vi "Live Image Test_cpattern match.vi"() -> ()   [LabVIEW 2017]
uses:
  <vilib>/vision/NI_Vision_Development_Module.lvlib
panel:
  in  "Minimum Score":sgl=700.0
  in  "Learn":bool
  in  "Test":enum16{"Color Pattern", "no test"}(ring)
  in  "Enum":T1(ring)
  in  "Acquire Params":T2={"fps"=10, "Compression"=30, "X"=320, "Y"=240, "Enable Color?"=TRUE, "Rotation"=enum."0"}
  out "Waveform Chart":u32(graph)
  out "dT":u32
  in  "stop":bool
  out "Image":T3(plugin-control)
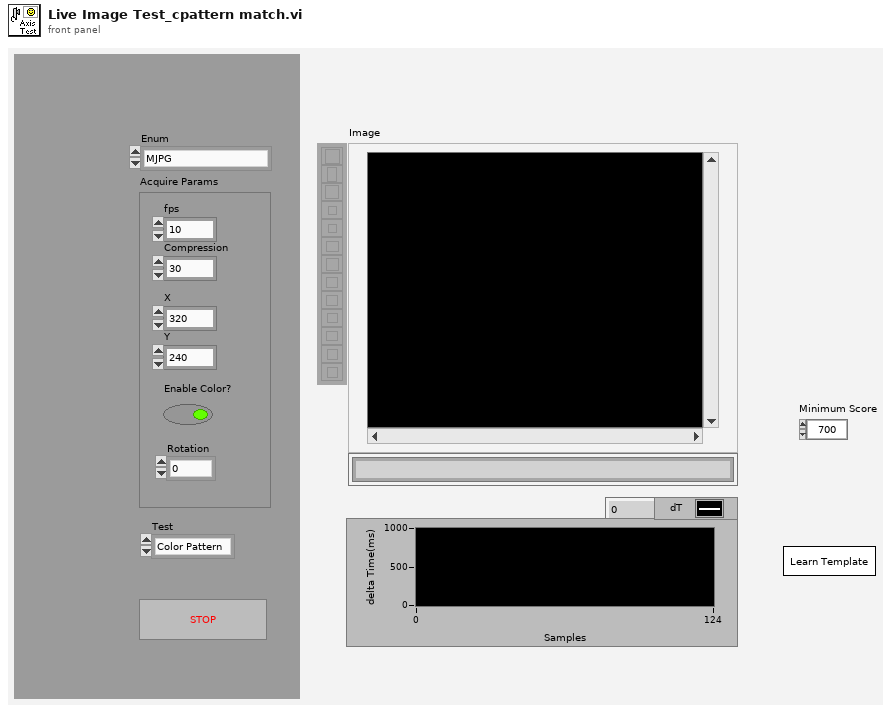
[diagram p1: front panel]
types:
  T1 = enum16{"MJPG", "JPG", "JPG-CGI", "BMP", "BMP-CGI"}
  T2 = cluster{"fps":i32, "Compression":i32, "X":i32, "Y":i32, "Enable Color?":bool, "Rotation":enum16{"0", "90", "180", "270"}}
  T3 = typedef "IMAQ Image.ctl" = refnum<image>
  T4 = typedef "Image Type" = u32
  T5 = cluster{"Global Rectangle":i32[], "Contours":cluster{"Contour Type":u32, "ROI Type":u32, "Points":i32[]}[]}
  T6 = cluster{i32[], cluster{"Contour Type":u32, "ROI Type":u32, i32[]}[]}
  T7 = cluster{"Position":cluster{"x":sgl, "y":sgl}, "Angle":sgl, "Scale":sgl, "Score":sgl, "Bounding Box":cluster{"x":sgl, "y":sgl}[]}[]
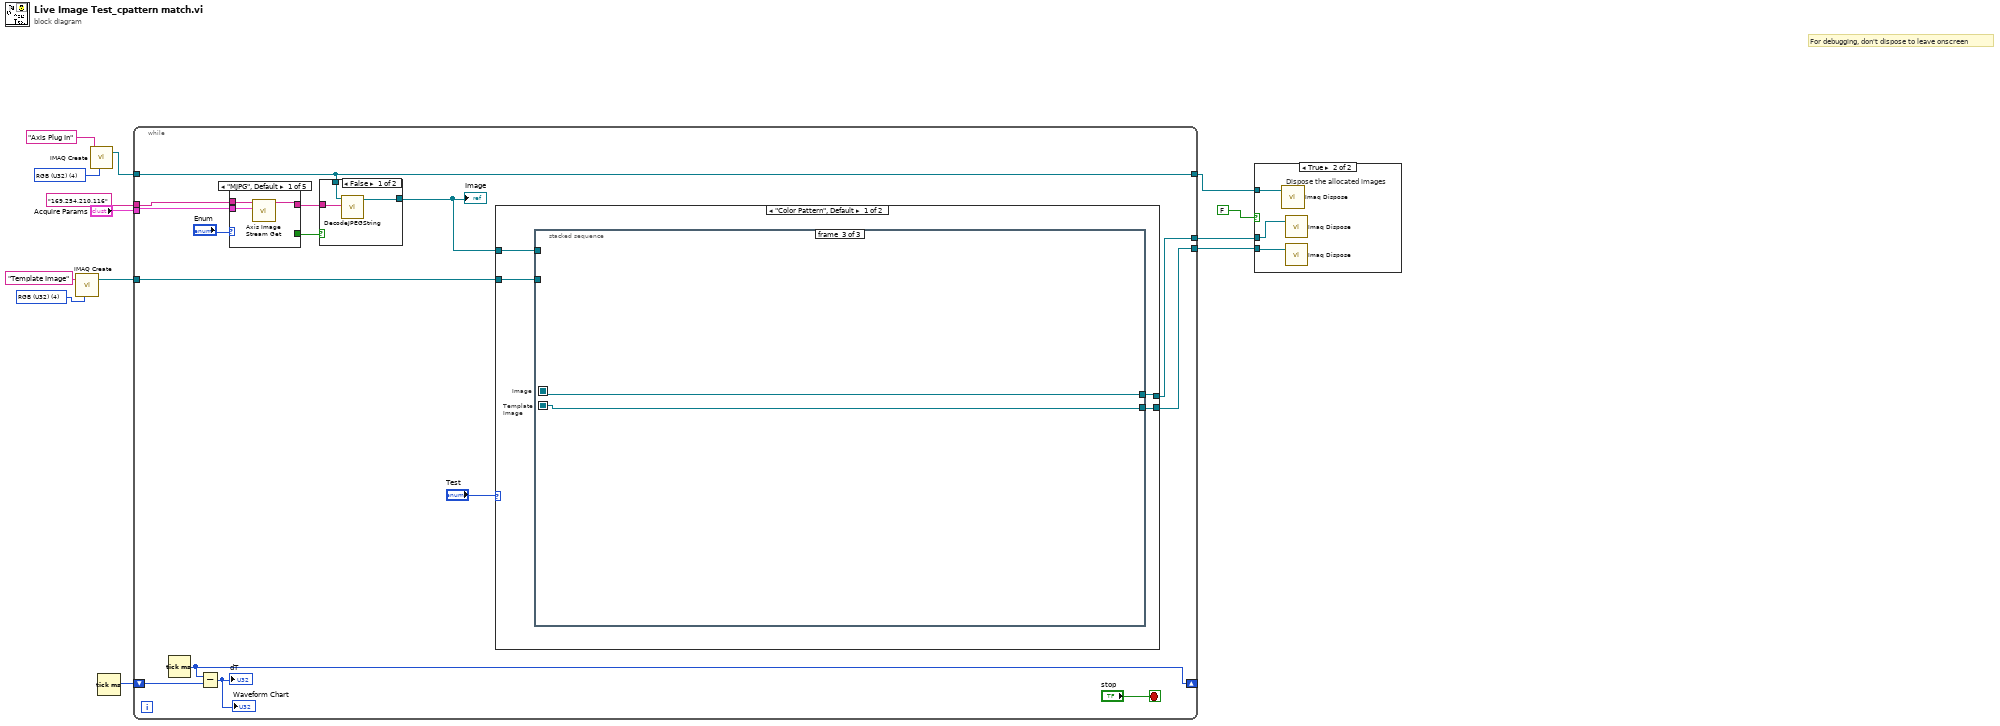
[diagram p0: block diagram]
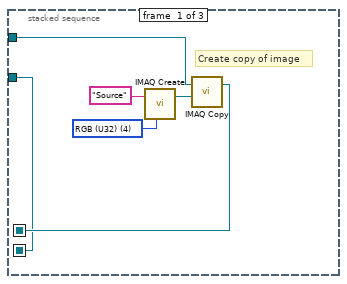
[diagram p3: hidden frame]
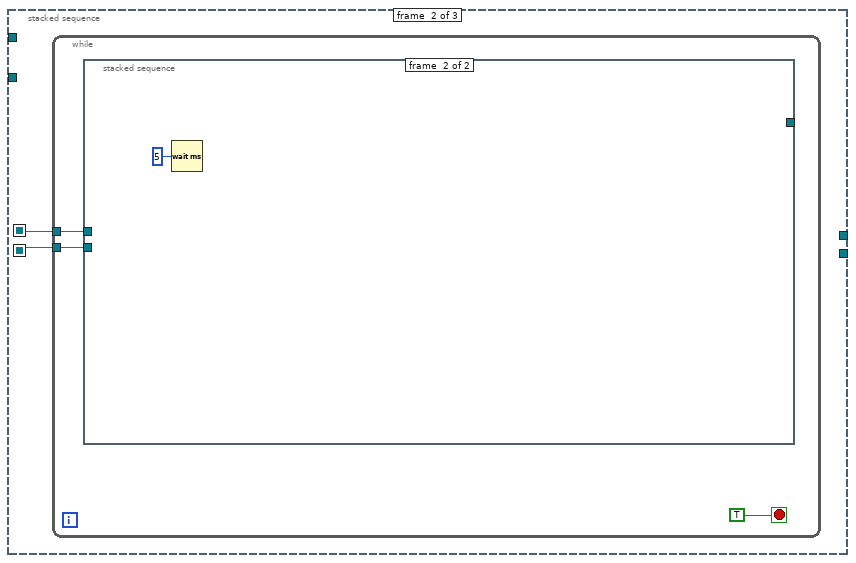
[diagram p4: hidden frame]
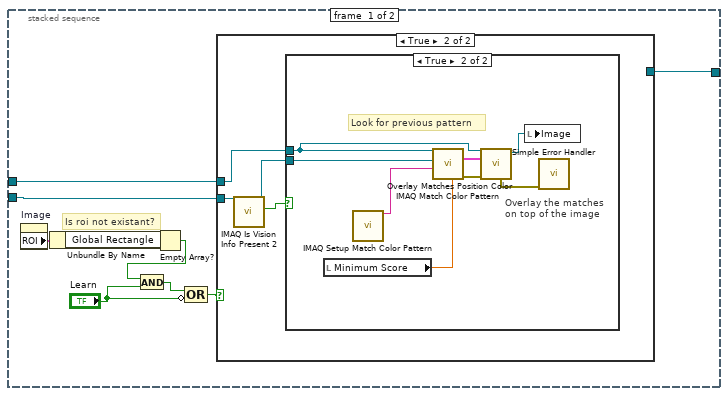
[diagram p5: hidden frame]
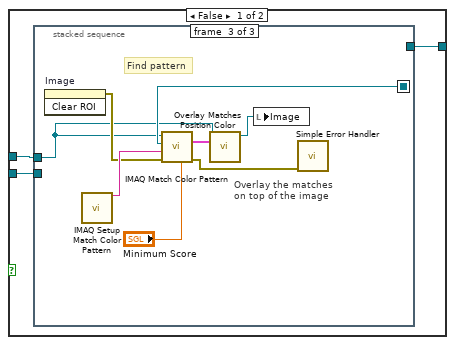
[diagram p6: hidden frame]
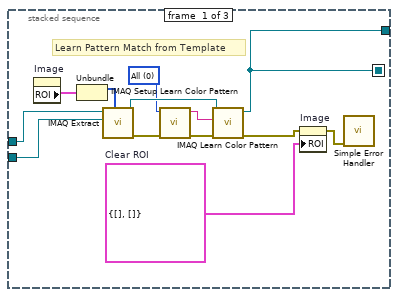
[diagram p7: hidden frame]
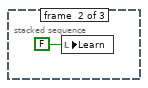
[diagram p8: hidden frame]
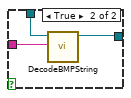
[diagram p11: hidden frame]
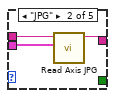
[diagram p12: hidden frame]
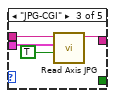
[diagram p13: hidden frame]
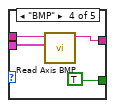
[diagram p14: hidden frame]
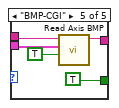
[diagram p15: hidden frame]
diagram:
  w5 = T4 4 items=["Grayscale (U8)", "Grayscale (I16)", "Grayscale (SGL)", "Complex (CSG)", "RGB (U32)", "HSL (U32)", "RGB (U64)", "Grayscale (U16)"] ("Image Type")
  w6 = T4 4 items=["Grayscale (U8)", "Grayscale (I16)", "Grayscale (SGL)", "Complex (CSG)", "RGB (U32)", "HSL (U32)", "RGB (U64)"] ("Image Type")
  # "For debugging, don't dispose to leave onscreen"
  n1 = call "IMAQ Create"("Image Name"="Template Image", "Image Type"=w5) -> ("New Image"=w3:T3)  [unwired: 3 in, 1 out]
  n2 = call "IMAQ Create"("Image Name"="Axis Plug In", "Image Type"=w6) -> ("New Image"=w12:T3)  [unwired: 3 in, 1 out]
  n3 = Tick Count (ms)() -> (millisecond timer value=w11:u32)
  n4 = while {
    tunnel: w12 -> [w24]
    shift-right: [w26] -> _
    shift-left: w11 -> [w27]
    tunnel: [w24] -> w10
    tunnel: "169.254.210.116" ("address") -> [w23]
    tunnel: "Acquire Params" -> [w20]
    tunnel: w3 -> [w17]
    tunnel: [w16] -> w2
    tunnel: [w15] -> w1
    stop <- "stop" stop-if-true
    n5 = Tick Count (ms)() -> (millisecond timer value=w26:u32)
    n6 = Subtract(x=w26, y=w27) -> (x-y=→"dT" →"Waveform Chart":u32)
    n7 = case shown="\"MJPG\", Default" "Enum" {
      tunnel: w23 -> [w100 w103 w107 w111 w115]
      tunnel: [w99 w102 w106 w110 w116] -> w22
      tunnel: w20 -> [w98 w101 w105 w109 w114]
      tunnel: [_ _ _ TRUE TRUE] -> w19
      frame "MJPG", Default {
        n8 = call <vilib>:"Axis Image Stream Get.vi"("Acquire Params"=w98, "IP Address"=w100) -> ("Raw Image Data"=w99:string)  [unwired: 9 in]
      }
      frame "JPG" {
        n9 = call <vilib>:"Read Axis JPG.vi"("Acquire Params"=w101, "address"=w103) -> ("Raw Image Data"=w102:string)  [unwired: 8 in, 1 out]
      }
      frame "JPG-CGI" {
        n10 = call <vilib>:"Read Axis JPG.vi"("CGI?"=TRUE, "Acquire Params"=w105, "address"=w107) -> ("Raw Image Data"=w106:string)  [unwired: 7 in, 1 out]
      }
      frame "BMP" {
        n11 = call <vilib>:"Read Axis BMP.vi"("Acquire Params"=w109, "address"=w111) -> ("Raw Image Data"=w110:string)  [unwired: 8 in, 1 out]
      }
      frame "BMP-CGI" {
        n12 = call <vilib>:"Read Axis BMP.vi"("CGI?"=TRUE, "Acquire Params"=w114, "address"=w115) -> ("Raw Image Data"=w116:string)  [unwired: 7 in, 1 out]
      }
    }
    n13 = case shown="False" w19 {
      tunnel: [w94 w96] -> w14
      tunnel: w24 -> [w93 w97]
      tunnel: w22 -> [w92 w95]
      frame False {
        n14 = call <vilib>:"DecodeJPEGString.vi"("Compressed Image"=w92, "Image In"=w93) -> ("Image Out"=w94:T3)  [unwired: 4 in, 1 out]
      }
      frame True {
        n15 = call <vilib>:"DecodeBMPString.vi"("Compressed Image"=w95, "Image In"=w97) -> ("Image Out"=w96:T3)  [unwired: 4 in, 1 out]
      }
    }
    "Image" <- w14
    n16 = case shown="\"Color Pattern\", Default" "Test" {
      tunnel: w17 -> [w32 _]
      tunnel: [w31 _] -> w16
      tunnel: [w30 _] -> w15
      tunnel: w14 -> [w29 _]
      frame "Color Pattern", Default {
        # "Template\nImage"
        # "Image"
        n17 = stacked-sequence {
          seq-local: [w36 _ _] -> [_ w39 w91]
          seq-local: [w34 _ _] -> [_ w40 w90]
          tunnel: w32 -> [w34 _ _]
          tunnel: [_ _ w91] -> w31
          tunnel: [_ _ w90] -> w30
          tunnel: w29 -> [w33 _ _]
          frame #0 {
            w35 = T4 4 items=["Grayscale (U8)", "Grayscale (I16)", "Grayscale (SGL)", "Complex (CSG)", "RGB (U32)", "HSL (U32)", "RGB (U64)", "Grayscale (U16)"] ("Image Type")
            # "Create copy of image"
            n18 = call "IMAQ Create"("Image Name"="Source", "Image Type"=w35) -> ("New Image"=w37:T3)  [unwired: 3 in, 1 out]
            n19 = call "IMAQ Copy"("Image Dst"=w37, "Image Src"=w33) -> ("Image Dst Out"=w36:T3)  [unwired: 4 in, 1 out]
          }
          frame #1 {
            n20 = while {
              tunnel: w40 -> [w43]
              tunnel: w39 -> [w42]
              stop <- TRUE stop-if-true
              n21 = stacked-sequence {
                tunnel: w43 -> [w52 _]
                tunnel: w42 -> [w51 _]
                tunnel: [w50 _] -> _
                frame #0 {
                  # "Is roi not existant?"
                  n22 = property on="Image" class="ImageControl"() -> ("ROI"=w48:T5)  [unwired: 2 in, 2 out]
                  n23 = Unbundle By Name(w48) -> ("Global Rectangle"=w49:i32[])
                  n24 = Empty Array?(array=w49) -> (empty?=w47:bool)
                  n25 = And(x=w47, y="Learn") -> (x .and. y?=w44:bool)
                  n26 = Compound Arithmetic op=OR(w44, invert "Learn") -> (w46:bool)
                  n27 = case shown="True" w46 {
                    tunnel: w52 -> [w53 w81]
                    tunnel: w51 -> [w55 w78]
                    tunnel: [w54 _] -> w50
                    frame False {
                      n28 = stacked-sequence {
                        seq-local: [w56 _ _] -> [_ _ w73]
                        tunnel: w53 -> [w66 _ _]
                        tunnel: w55 -> [w57 _ w71]
                        tunnel: [w56 _ _] -> w54
                        frame #0 {
                          w62 = u32 0 items=["All", "Shift Information", "Rotation Information"] ("Learn Mode")
                          w60 = T6 {[], []}  # Clear ROI
                          # "Learn Pattern Match from Template"
                          n29 = property on="Image" class="ImageControl"() -> ("ROI"=w61:T5)  [unwired: 2 in, 2 out]
                          n30 = Unbundle(w61) -> ("Global Rectangle"=w68:i32[])  [unwired: 1 out]
                          n31 = call "IMAQ Extract"("Optional Rectangle"=w68, "Image Dst"=w66, "Image Src"=w57) -> ("error out"=w64:errorcluster, "Image Dst Out"=w65:T3)  [unwired: 7 in]
                          n32 = call "IMAQ Setup Learn Color Pattern"("error in (no error)"=w64, "Learn Mode"=w62) -> ("error out"=w63:errorcluster, "Learn Color Pattern Setup Data"=w67:string)  [unwired: 8 in]
                          n33 = call "IMAQ Learn Color Pattern"("error in (no error)"=w63, "Learn Color Pattern Setup Data"=w67, "Image"=w65) -> ("error out"=w59:errorcluster, "Template Image Out"=w56:T3)  [unwired: 7 in]
                          n34 = property on="Image" class="ImageControl"(error in=w59, "ROI"=w60) -> (error out=w58:errorcluster)  [unwired: 1 in, 1 out]
                          n35 = call <vilib>:"Simple Error Handler.vi"("error in (no error)"=w58) -> ()  [unwired: 4 in, 5 out]
                        }
                        frame #1 {
                          n36 = local write "Learn"(FALSE ("Blinking")) -> ()
                        }
                        frame #2 {
                          # "Find pattern"
                          # "Overlay the matches on top of the image"
                          n37 = invoke on="Image" class="ImageControl" method="Clear ROI"() -> (error out=w72:errorcluster)  [unwired: 3 in, 2 out]
                          n38 = call "IMAQ Setup Match Color Pattern"() -> ("Match Color Pattern Setup Data"=w77:string)  [unwired: 14 in, 1 out]
                          n39 = call "IMAQ Match Color Pattern"("Minimum Match Score"="Minimum Score", "error in (no error)"=w72, "Match Color Pattern Setup Data"=w77, "Template Image"=w73, "Image"=w71) -> ("error out"=w74:errorcluster, "Matches"=w75:T7)  [unwired: 4 in, 1 out]
                          n40 = call "Overlay Matches Position Color.vi"("Matches"=w75, "Image"=w71) -> ("Image Out"=w70:T3)  [unwired: 9 in]
                          n41 = local write "Image"(w70) -> ()
                          n42 = call <vilib>:"Simple Error Handler.vi"("error in (no error)"=w74) -> ()  [unwired: 4 in, 5 out]
                        }
                      }
                    }
                    frame True {
                      n43 = call "IMAQ Is Vision Info Present 2"("Image"=w81) -> ("Present?"=w80:bool, "Image (duplicate)"=w79:T3)  [unwired: 8 in, 1 out]
                      n44 = case shown="True" w80 {
                        tunnel: w79 -> [_ w83]
                        tunnel: w78 -> [_ w82]
                        frame False {
                        }
                        frame True {
                          # "Look for previous pattern"
                          # "Overlay the matches on top of the image"
                          n45 = local read "Minimum Score"() -> (w84:sgl)
                          n46 = call "IMAQ Setup Match Color Pattern"() -> ("Match Color Pattern Setup Data"=w88:string)  [unwired: 14 in, 1 out]
                          n47 = call "IMAQ Match Color Pattern"("Minimum Match Score"=w84, "Match Color Pattern Setup Data"=w88, "Template Image"=w83, "Image"=w82) -> ("error out"=w86:errorcluster, "Matches"=w87:T7)  [unwired: 5 in, 1 out]
                          n48 = call "Overlay Matches Position Color.vi"("Matches"=w87, "Image"=w82) -> ("Image Out"=w85:T3)  [unwired: 9 in]
                          n49 = local write "Image"(w85) -> ()
                          n50 = call <vilib>:"Simple Error Handler.vi"("error in (no error)"=w86) -> ()  [unwired: 4 in, 5 out]
                        }
                      }
                    }
                  }
                }
                frame #1 {
                  n51 = Wait (ms)(milliseconds to wait=u32 5) -> ()  [unwired: 1 out]
                }
              }
            }
          }
          frame #2 {
          }
        }
      }
      frame "no test" {
      }
    }
  }
  n52 = case shown="True" FALSE {
    tunnel: w10 -> [_ w119]
    tunnel: w2 -> [_ w118]
    tunnel: w1 -> [_ w117]
    frame False {
    }
    frame True {
      # "Dispose the allocated images"
      n53 = call "Imaq Dispose"("Image"=w119) -> ()  [unwired: 5 in, 1 out]
      n54 = call "Imaq Dispose"("Image"=w118) -> ()  [unwired: 5 in, 1 out]
      n55 = call "Imaq Dispose"("Image"=w117) -> ()  [unwired: 5 in, 1 out]
    }
  }
